vi "HeartSoundPeakDetect.vi"(4 "Max time to peak\nfrom threshold (ms)":dbl, 6 "Min time between\nbeats (ms)":dbl, 9 "width (threshold)":i32, 10 "Threshold multiplier":dbl, 11 "Sound":waveform(dbl)) -> (0 "Threshold":dbl, 2 "Peaks Y":dbl[](array[numeric]), 3 "Peaks X":dbl[](array[numeric]))   [LabVIEW 2014, in "Phonocardiography.lvlib"]
uses:
  Phonocardiography.lvlib
  <vilib>/Waveform/WDTOps.llb/WDT Get Waveform Time Array DBL.vi
  <vilib>/Analysis/NI_AALPro.lvlib
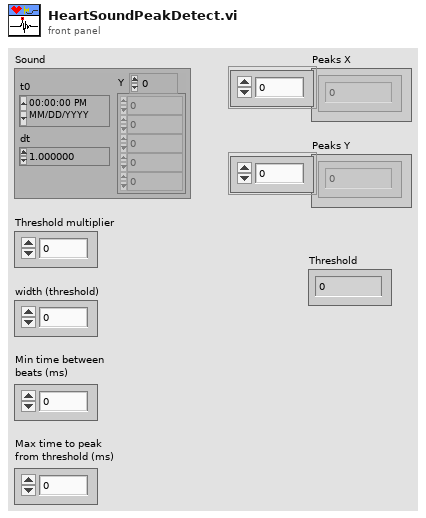
[diagram p1: front panel]
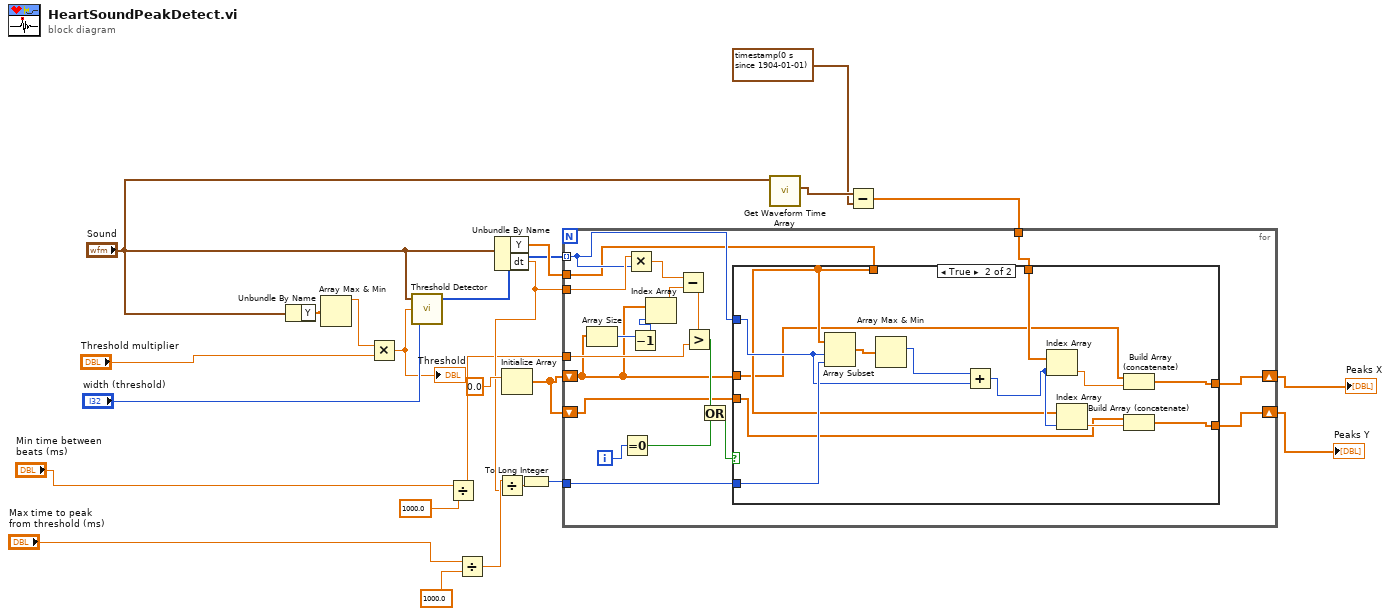
[diagram p0: block diagram]
diagram:
  n1 = Unbundle By Name("Sound") -> ("Y"=w6:dbl[])
  n2 = Array Max & Min(array=w6) -> (max value=w5:dbl)  [unwired: 3 out]
  n3 = Multiply(x=w5, y="Threshold multiplier") -> (x*y=w10:dbl)
  "Threshold" <- w10
  n4 = call <vilib>:"Threshold Detector.vi"("width"="width (threshold)", "threshold"=w10, "X"="Sound") -> ("Indices"=w12:i32[])  [unwired: 2 out]
  n5 = Divide(x="Min time between\nbeats (ms)", y=1000.0) -> (x/y=w13:dbl)
  n6 = Divide(x="Max time to peak\nfrom threshold (ms)", y=1000.0) -> (x/y=w19:dbl)
  n7 = Unbundle By Name("Sound") -> ("Y"=w22:dbl[], "dt"=w14:dbl)
  n8 = Divide(x=w19, y=w14) -> (x/y=w15:dbl)
  n9 = Initialize Array(0.0 ("y")) -> (w23:dbl[])  [unwired: 1 in]
  n10 = To Long Integer(number=w15) -> (32bit integer=w16:i32)
  n11 = call-poly <vilib>:"Get Waveform Time Array.vi"("waveform in"="Sound") -> ("X array"=w4:timestamp[])  [unwired: 9 in, 1 out]
  n12 = Subtract(x=w4, y=timestamp(0 s since 1904-01-01) ("Xo")) -> (x-y=w2:dbl[])
  n13 = for {
    tunnel: w12 -> [w31] mode=indexing
    tunnel: w22 -> [w30]
    tunnel: w14 -> [w43]
    tunnel: w13 -> [w40]
    tunnel: w16 -> [w32]
    shift-right: [w29] -> w24
    shift-left: w23 -> [w25]
    shift-right: [w27] -> w21
    shift-left: w23 -> [w28]
    tunnel: w2 -> [w26]
    i -> [w39]
    n14 = Array Size(array=w25) -> (size(s)=w35:i32)
    n15 = Equal To 0?(x=w39) -> (x = 0?=w38:bool)
    n16 = Multiply(x=w43, y=w31) -> (x*y=w42:dbl)
    n17 = Decrement(x=w35) -> (x-1=w34:i32)
    n18 = Index Array(array=w25, index=w34) -> (element=w33:dbl)
    n19 = Subtract(x=w42, y=w33) -> (x-y=w41:dbl)
    n20 = Greater?(x=w41, y=w40) -> (0:w37:bool)
    n21 = Or(x=w37, y=w38) -> (x .or. y?=w36:bool)
    n22 = case shown="True" w36 {
      tunnel: w32 -> [_ w58]
      tunnel: w31 -> [_ w55]
      tunnel: w30 -> [_ w52]
      tunnel: w25 -> [w45 w48]
      tunnel: [w45 w47] -> w29
      tunnel: w28 -> [w44 w49]
      tunnel: [w44 w46] -> w27
      tunnel: w26 -> [_ w53]
      frame False {
      }
      frame True {
        n23 = Array Subset(array=w52, index=w55, length=w58) -> (w57:dbl[])
        n24 = Array Max & Min(array=w57) -> (max index (indices)=w56:i32)  [unwired: 3 out]
        n25 = Add(x=w56, y=w55) -> (x+y=w54:i32)
        n26 = Index Array(array=w53, index=w54) -> (element=w51:dbl)
        n27 = Index Array(array=w52, index=w54) -> (element=w50:dbl)
        n28 = Build Array (concatenate)(w48, w51) -> (w47:dbl[])
        n29 = Build Array (concatenate)(w49, w50) -> (w46:dbl[])
      }
    }
  }
  "Peaks X" <- w24
  "Peaks Y" <- w21
